vi "_builtins_arrange_constant.vi"(8 "error in (no error)":errorcluster, 11 "GObject in":refnum<vi>) -> (0 "error out":errorcluster, 2 "object arranged?":bool, 3 "GObject out":refnum<vi>)   [LabVIEW 2019, in "Script.lvlib"]
doc: "Arranges the constant relative to the terminal position.\n\nCreated by: Ryan Pacini"
uses:
  Script.lvlib
  <vilib>/Utility/miscctls.llb/LVPositionTypeDef.ctl
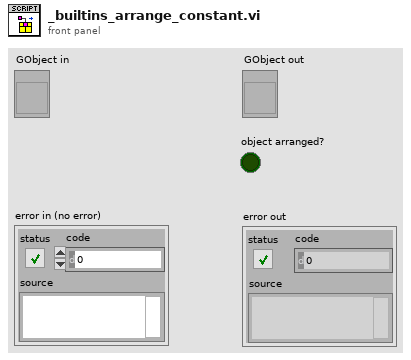
[diagram p1: front panel]
types:
  T1 = typedef "LVPositionTypeDef.ctl" = cluster{"Left":i32, "Top":i32}
  T2 = typedef "LVRectTypeDef.ctl" = cluster{"Left":i16, "Top":i16, "Right":i16, "Bottom":i16}
  T3 = cluster{"Left":i32, "Top":i32, "Right":i32, "Bottom":i32}
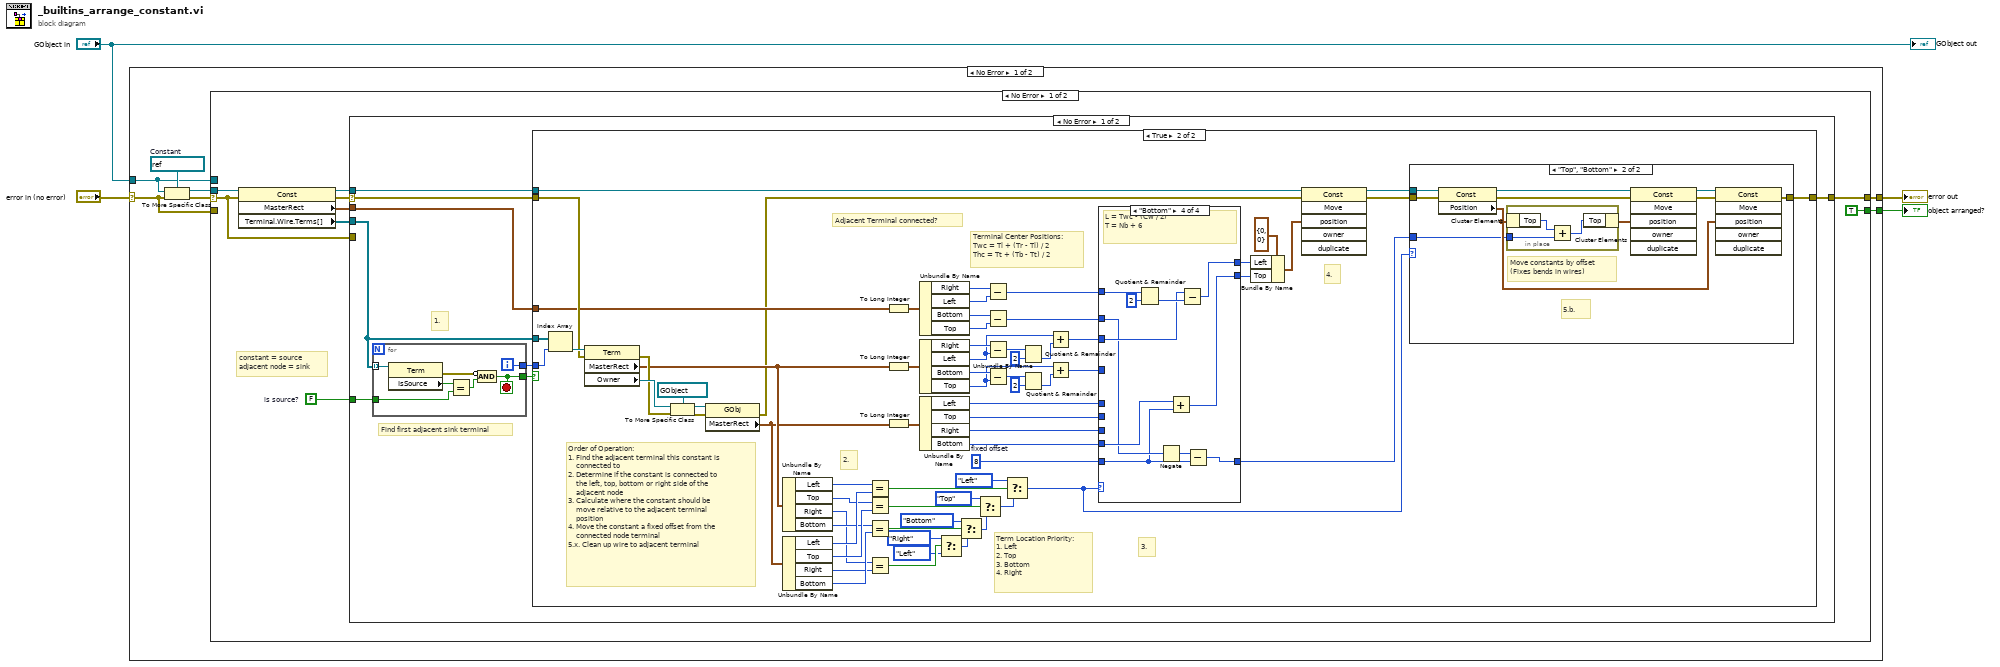
[diagram p0: block diagram]
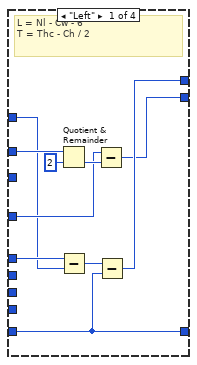
[diagram p3: hidden frame]
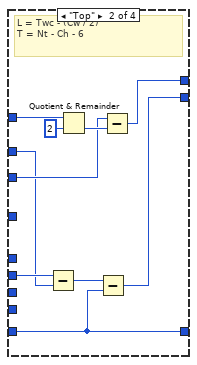
[diagram p4: hidden frame]
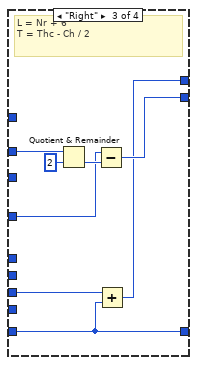
[diagram p5: hidden frame]
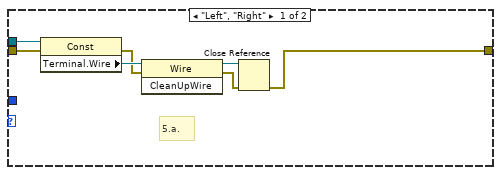
[diagram p6: hidden frame]
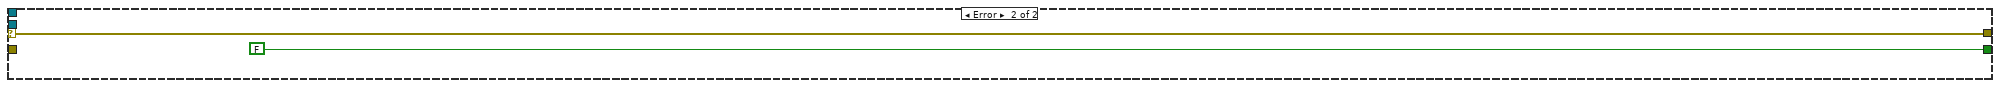
[diagram p8: hidden frame]
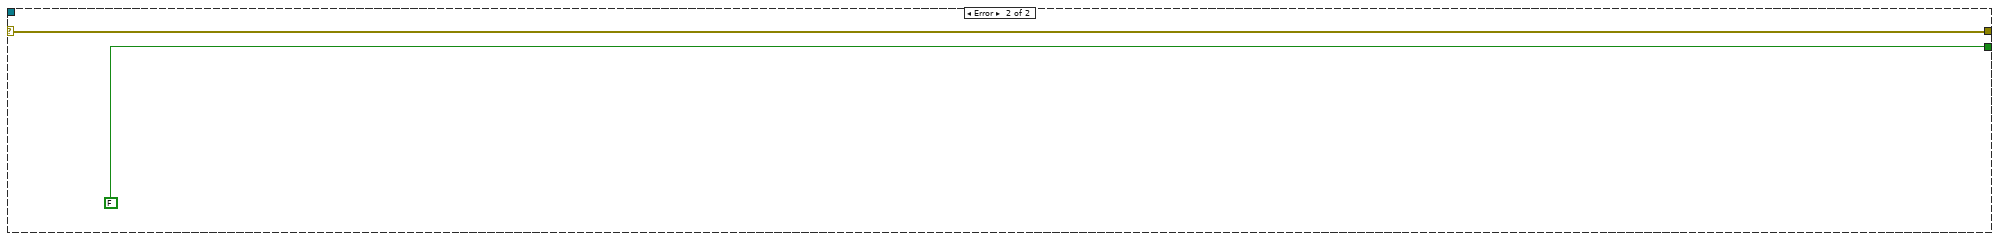
[diagram p9: hidden frame]
diagram:
  n1 = case shown="No Error" "error in (no error)" {
    selector: "error in (no error)" -> [w5 w169]
    tunnel: "GObject in" -> [w6 _]
    tunnel: [w11 w169] -> w2
    tunnel: [w10 FALSE] -> w1
    frame No Error {
      w9 = refnum<vi> refnum  # Constant
      n2 = To More Specific Class(target class=w9, reference=w6, error in=w5) -> (specific class reference=w7:refnum<vi>, error out=w8:errorcluster)
      n3 = case shown="No Error" w8 {
        selector: w8 -> [w12 _]
        tunnel: w7 -> [w19 _]
        tunnel: w6 -> [_ _]
        tunnel: w5 -> [_ w167]
        tunnel: [w15 w167] -> w11
        tunnel: [TRUE FALSE] -> w10
        frame No Error {
          w17 = FALSE  # is source?
          # "constant = source\nadjacent node = sink"
          n4 = property class="Const"(reference=w19, error in=w12) -> (reference out=w14:refnum<vi>, error out=w13:errorcluster, "MasterRect"=w16:T2, "Terminal.Wire.Terms[]"=w18:refnum<vi>[])
          n5 = case shown="No Error" w13 {
            selector: w13 -> [w21 _]
            tunnel: w18 -> [w28 _]
            tunnel: w17 -> [w27 _]
            tunnel: w16 -> [w24 _]
            tunnel: [w23 w165] -> w15
            tunnel: w14 -> [w22 _]
            tunnel: w12 -> [_ w165]
            frame No Error {
              # "1."
              # "Find first adjacent sink terminal"
              n6 = for {
                tunnel: w28 -> [w164] mode=indexing
                tunnel: [w163] -> w25
                tunnel: [w161] -> w26
                tunnel: w27 -> [w159]
                i -> [w163]
                stop <- w161 stop-if-true
                n7 = property class="Term"(reference=w164) -> (error out=w162:errorcluster, "IsSource"=w160:bool)  [unwired: 1 in, 1 out]
                n8 = Equal?(x=w160, y=w159) -> (x = y?=w158:bool)
                n9 = Compound Arithmetic op=AND(invert w162, w158) -> (w161:bool)
              }
              n10 = case shown="True" w26 {
                tunnel: w28 -> [_ w96]
                tunnel: w25 -> [_ w91]
                tunnel: w21 -> [w29 w90]
                tunnel: w24 -> [_ w69]
                tunnel: [w29 w35] -> w23
                tunnel: w22 -> [_ w37]
                frame False {
                }
                frame True {
                  w51 = 8  # fixed offset
                  # "Terminal Center Positions:\nTwc = Tl + (Tr - Tl) / 2\nThc = Tt + (Tb - Tt) / 2"
                  # "Order of Operation:\n1. Find the adjacent terminal this constant is \n    connected to\n2. Determine if the constant is connected to \n    the left, top, bottom or right side of the \n    adjacent node\n3. Calculate where the constant should be \n    move relative to the adjacent terminal\n    position\n4. Move the constant a fixed offset from the\n    connected node terminal \n5.x. Clean up wire to adjacent terminal"
                  # "4."
                  # "3."
                  # "2."
                  # "Term Location Priority:\n1. Left\n2. Top\n3. Bottom\n4. Right"
                  # "Adjacent Terminal connected?"
                  n11 = Index Array(array=w96, index=w91) -> (element=w98:refnum<vi>)
                  n12 = property class="Term"(reference=w98, error in=w90) -> (error out=w94:errorcluster, "MasterRect"=w58:T2, "Owner"=w97:refnum<vi>)  [unwired: 1 out]
                  n13 = To More Specific Class(target class=refnum<vi> refnum ("Owner"), reference=w97, error in=w94) -> (specific class reference=w95:refnum<vi>, error out=w92:errorcluster)
                  n14 = property class="GObj"(reference=w95, error in=w92) -> (error out=w36:errorcluster, "MasterRect"=w56:T2)  [unwired: 1 out]
                  n15 = Unbundle By Name(w58) -> ("Left"=w89:i16, "Top"=w87:i16, "Right"=w75:i16, "Bottom"=w78:i16)
                  n16 = Unbundle By Name(w56) -> ("Left"=w88:i16, "Top"=w86:i16, "Right"=w74:i16, "Bottom"=w76:i16)
                  n17 = Equal?(x=w89, y=w88) -> (x = y?=w85:bool)
                  n18 = Equal?(x=w87, y=w86) -> (x = y?=w81:bool)
                  n19 = Equal?(x=w78, y=w76) -> (x = y?=w77:bool)
                  n20 = Equal?(x=w75, y=w74) -> (x = y?=w72:bool)
                  n21 = To Long Integer(number=w69) -> (32bit integer=w66:T3)
                  n22 = To Long Integer(number=w58) -> (32bit integer=w60:T3)
                  n23 = To Long Integer(number=w56) -> (32bit integer=w57:T3)
                  n24 = Unbundle By Name(w66) -> ("Right"=w67:i32, "Left"=w68:i32, "Bottom"=w65:i32, "Top"=w64:i32)
                  n25 = Unbundle By Name(w60) -> ("Right"=w59:i32, "Left"=w39:i32, "Bottom"=w61:i32, "Top"=w38:i32)
                  n26 = Unbundle By Name(w57) -> ("Left"=w55:i32, "Top"=w54:i32, "Right"=w53:i32, "Bottom"=w52:i32)
                  n27 = Select(t=enum8{"Left", "Top", "Right", "Bottom"}."Right" ("Location"), s=w72, f=enum8{"Left", "Top", "Right", "Bottom"}."Left" ("Location")) -> (s? t:f=w71:enum8{"Left", "Top", "Right", "Bottom"})
                  n28 = Select(t=enum8{"Left", "Top", "Right", "Bottom"}."Bottom" ("Location"), s=w77, f=w71) -> (s? t:f=w79:enum8{"Left", "Top", "Right", "Bottom"})
                  n29 = Select(t=enum8{"Left", "Top", "Right", "Bottom"}."Top" ("Location"), s=w81, f=w79) -> (s? t:f=w82:enum8{"Left", "Top", "Right", "Bottom"})
                  n30 = Subtract(x=w67, y=w68) -> (x-y=w63:i32)
                  n31 = Subtract(x=w65, y=w64) -> (x-y=w62:i32)
                  n32 = Subtract(x=w59, y=w39) -> (x-y=w44:i32)
                  n33 = Subtract(x=w61, y=w38) -> (x-y=w41:i32)
                  n34 = Select(t=enum8{"Left", "Top", "Right", "Bottom"}."Left" ("Location"), s=w85, f=w82) -> (s? t:f=w33:enum8{"Left", "Top", "Right", "Bottom"})
                  n35 = Quotient & Remainder(x=w44, y=2) -> (floor(x/y)=w45:i32)  [unwired: 1 out]
                  n36 = Quotient & Remainder(x=w41, y=2) -> (floor(x/y)=w32:i32)  [unwired: 1 out]
                  n37 = Add(x=w39, y=w45) -> (x+y=w43:i32)
                  n38 = Add(x=w38, y=w32) -> (x+y=w40:i32)
                  n39 = case shown="\"Bottom\"" w33 {
                    tunnel: [w101 w112 w120 w137] -> w50
                    tunnel: [w100 w113 w121 w132] -> w49
                    tunnel: w63 -> [w103 w117 _ w135]
                    tunnel: w62 -> [w106 w110 w124 w130]
                    tunnel: w43 -> [_ w111 _ w133]
                    tunnel: w40 -> [w105 _ w123 _]
                    tunnel: w55 -> [w104 _ _ _]
                    tunnel: w54 -> [_ w115 _ _]
                    tunnel: w53 -> [_ _ w122 _]
                    tunnel: w52 -> [_ _ _ w131]
                    tunnel: w51 -> [w99 w109 w119 w127]
                    tunnel: [w99 w109 w119 w129] -> w34
                    frame "Left" {
                      # "L = Nl - Cw - 6\nT = Thc - Ch / 2"
                      n40 = Quotient & Remainder(x=w106, y=2) -> (floor(x/y)=w107:i32)  [unwired: 1 out]
                      n41 = Subtract(x=w104, y=w103) -> (x-y=w102:i32)
                      n42 = Subtract(x=w105, y=w107) -> (x-y=w100:i32)
                      n43 = Subtract(x=w102, y=w99) -> (x-y=w101:i32)
                    }
                    frame "Top" {
                      # "L = Twc - (Cw / 2)\nT = Nt - Ch - 6"
                      n44 = Subtract(x=w115, y=w110) -> (x-y=w114:i32)
                      n45 = Quotient & Remainder(x=w117, y=2) -> (floor(x/y)=w116:i32)  [unwired: 1 out]
                      n46 = Subtract(x=w114, y=w109) -> (x-y=w113:i32)
                      n47 = Subtract(x=w111, y=w116) -> (x-y=w112:i32)
                    }
                    frame "Right" {
                      # "L = Nr + 6\nT = Thc - Ch / 2"
                      n48 = Quotient & Remainder(x=w124, y=2) -> (floor(x/y)=w125:i32)  [unwired: 1 out]
                      n49 = Subtract(x=w123, y=w125) -> (x-y=w121:i32)
                      n50 = Add(x=w122, y=w119) -> (x+y=w120:i32)
                    }
                    frame "Bottom" {
                      # "L = Twc - (Cw / 2)\nT = Nb + 6"
                      n51 = Quotient & Remainder(x=w135, y=2) -> (floor(x/y)=w134:i32)  [unwired: 1 out]
                      n52 = Negate(x=w130) -> (-x=w128:i32)
                      n53 = Add(x=w131, y=w127) -> (x+y=w132:i32)
                      n54 = Subtract(x=w133, y=w134) -> (x-y=w137:i32)
                      n55 = Subtract(x=w128, y=w127) -> (x-y=w129:i32)
                    }
                  }
                  n56 = Bundle By Name(cluster=T1 {"Left"=0, "Top"=0} ("Position"), "Left"=w50, "Top"=w49) -> (w47:T1)
                  n57 = invoke class="Const" method="Move"(reference=w37, error in=w36, "position"=w47) -> (reference out=w30:refnum<vi>, error out=w31:errorcluster)  [unwired: 3 in, 4 out]
                  n58 = case shown="\"Top\", \"Bottom\"" w33 {
                    tunnel: w30 -> [w141 w154]
                    tunnel: w31 -> [w138 w145]
                    tunnel: [w139 w150] -> w35
                    tunnel: w34 -> [_ w147]
                    frame "Left", "Right" {
                      # "5.a."
                      n59 = property class="Const"(reference=w141, error in=w138) -> (error out=w140:errorcluster, "Terminal.Wire"=w144:refnum<vi>)  [unwired: 1 out]
                      n60 = invoke class="Wire" method="CleanUpWire"(reference=w144, error in=w140) -> (reference out=w143:refnum<vi>, error out=w142:errorcluster)  [unwired: 1 in, 1 out]
                      n61 = Close Reference(reference=w143, error in (no error)=w142) -> (error out=w139:errorcluster)
                    }
                    frame "Top", "Bottom" {
                      # "5.b."
                      # "Move constants by offset\n(Fixes bends in wires)"
                      n62 = property class="Const"(reference=w154, error in=w145) -> (reference out=w153:refnum<vi>, error out=w152:errorcluster, "Position"=w148:T1)
                      n63 = in-place {
                        in-place-border: w147 -> [w155]
                        n64 = in-place-cluster #1(w148) -> ("Top"=w157:i32)
                        n65 = Add(x=w157, y=w155) -> (x+y=w156:i32)
                        n66 = in-place-cluster #1("Top"=w156) -> (w151:T1)
                      }
                      n67 = invoke class="Const" method="Move"(reference=w153, error in=w152, "position"=w151) -> (reference out=w149:refnum<vi>, error out=w146:errorcluster)  [unwired: 3 in, 4 out]
                      n68 = invoke class="Const" method="Move"(reference=w149, error in=w146, "position"=w148) -> (error out=w150:errorcluster)  [unwired: 3 in, 5 out]
                    }
                  }
                }
              }
            }
            frame Error {
              # "No wires connected"
            }
          }
        }
        frame Error {
        }
      }
    }
    frame Error {
    }
  }
  "error out" <- w2
  "object arranged?" <- w1
  "GObject out" <- "GObject in"
